vi "move-and-measure_v1.vi"(0 "meter-visa":refnum<visa-resource-name>, 1 "XY-in":dbl[](array[numeric]), 2 "bar-note":u8, 5 "PD Values":cluster{"PD1":dbl, "PD2":dbl, "PD3":dbl}, 7 "stage-refs":T1, 9 "meter-error-in":errorcluster, 11 "stage-error-in":errorcluster, 12 "counter-in":dbl format="%#_13g", 13 "meas#":dbl) -> (3 "measured-point out":dbl[](array[numeric]), 4 "logfile-line-out":string, 6 "iCorr-out":dbl, 10 "meter-error-out":errorcluster, 14 "counter-out":dbl, 15 "stage-error-out":errorcluster)   [LabVIEW 2024]
uses:
  C:/Users/hpDIRC/Desktop/eic_dirc_daq-LabVIEW_new/Thorlabs.MotionControl.IntegratedStepperMotorsCLI.dll
  Thorlabs.MotionControl.IntegratedStepperMotorsCLI.dll
  C:/Users/hpDIRC/Desktop/eic_dirc_daq-LabVIEW_new/Thorlabs.MotionControl.Benchtop.StepperMotorCLI.dll
  Thorlabs.MotionControl.Benchtop.StepperMotorCLI.dll
panel:
  in  "nSamples":dbl=10.0 caption="# Samples"
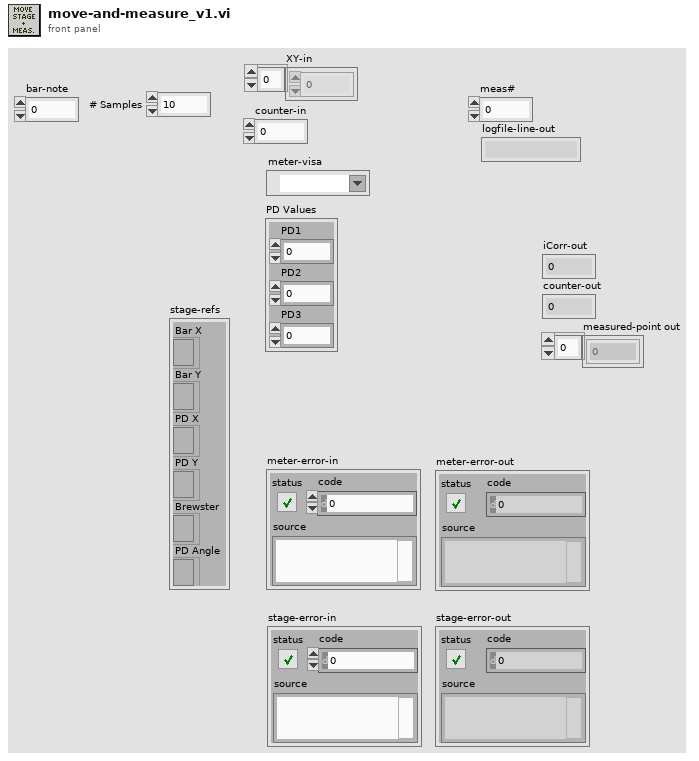
[diagram p1: front panel]
types:
  T1 = cluster{"Bar X":refnum<k24>, "Bar Y":refnum<k24>, "PD X":refnum<k24>, "PD Y":refnum<k24>, "Brewster":refnum<k24>, "PD Angle":refnum<k24>}
  T2 = cluster{"Bar X":dbl, "Bar Y":dbl, "PD X":dbl, "PD Y":dbl, "BMA":dbl, "PDA":dbl}
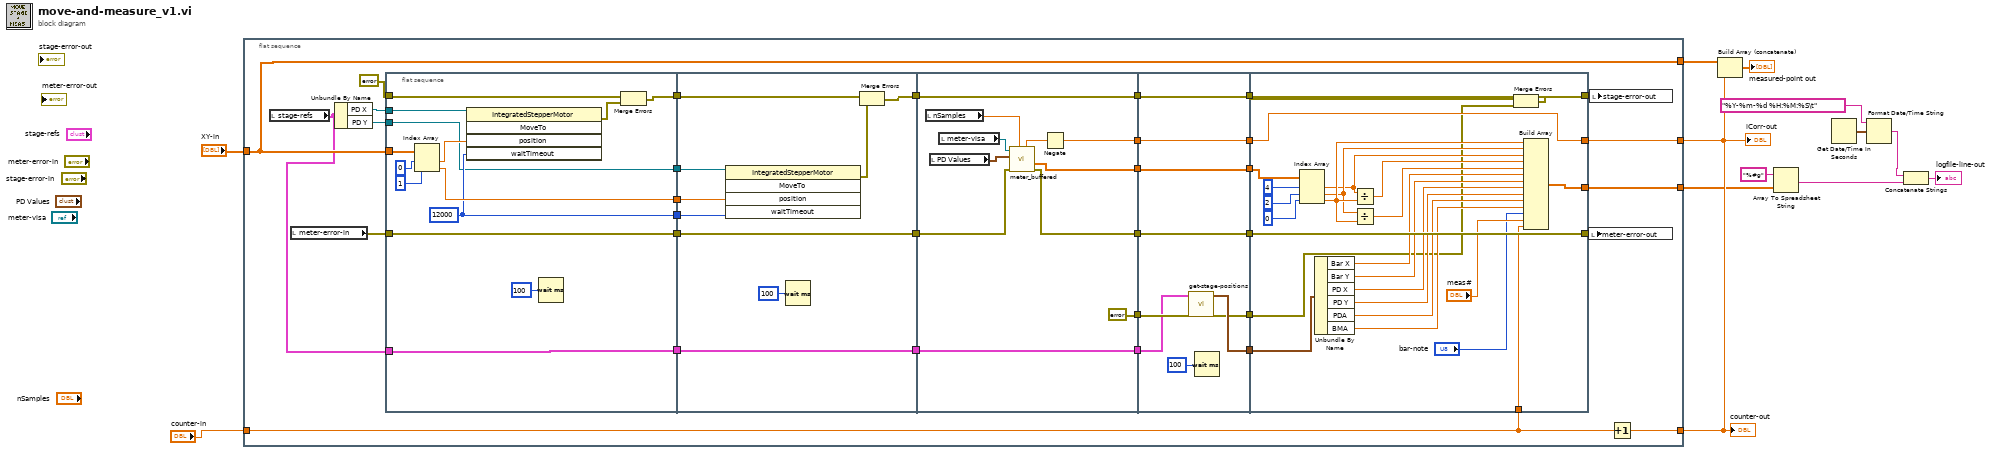
[diagram p0: block diagram]
diagram:
  n1 = flat-sequence {
    tunnel: [w45] -> w9
    tunnel: "XY-in" -> [w41]
    tunnel: "counter-in" -> [w38]
    tunnel: [w39] -> w8
    tunnel: [w41] -> w10
    tunnel: [w37] -> w5
    frame #0 {
      n2 = local read "stage-refs"() -> (w40:T1)
      n3 = local read "meter-error-in"() -> (w42:errorcluster)
      n4 = Unbundle By Name(w40) -> ("PD X"=w46:refnum<k24>, "PD Y"=w16:refnum<k24>)
      n5 = flat-sequence {
        tunnel: w46 -> [w59]
        tunnel: errorcluster {"status"=FALSE, "code"=0, "source"=""} ("stage-error-in") -> [w55]
        tunnel: w41 -> [w53]
        tunnel: w42 -> [w52]
        tunnel: [w54] -> w24
        tunnel: [w52] -> w22
        tunnel: [w51] -> w20
        tunnel: w40 -> [w51]
        tunnel: [w50] -> w18
        tunnel: [w49] -> w17
        tunnel: w16 -> [w48]
        tunnel: [w48] -> w15
        tunnel: w24 -> [w69]
        tunnel: [w63] -> w23
        tunnel: w22 -> [w68]
        tunnel: [w68] -> w21
        tunnel: w20 -> [w67]
        tunnel: [w67] -> w19
        tunnel: w18 -> [w66]
        tunnel: w17 -> [w65]
        tunnel: w15 -> [w64]
        tunnel: w23 -> [w71]
        tunnel: w21 -> [w79]
        tunnel: [w74] -> w36
        tunnel: [w78] -> w34
        tunnel: [w71] -> w32
        tunnel: [w73] -> w30
        tunnel: [w72] -> w28
        tunnel: w19 -> [w72]
        tunnel: [errorcluster {"status"=FALSE, "code"=0, "source"=""} ("error IO")] -> w26
        tunnel: w36 -> [w89]
        tunnel: [w89] -> w35
        tunnel: w34 -> [w88]
        tunnel: [w88] -> w33
        tunnel: w32 -> [w87]
        tunnel: [w87] -> w31
        tunnel: w30 -> [w86]
        tunnel: [w86] -> w29
        tunnel: w28 -> [w81]
        tunnel: [w83] -> w27
        tunnel: w26 -> [w85]
        tunnel: [w82] -> w25
        tunnel: [w91] -> w43
        tunnel: [w114] -> w44
        tunnel: [w96] -> w45
        tunnel: w35 -> [w96]
        tunnel: w33 -> [w114]
        tunnel: w31 -> [w90]
        tunnel: w29 -> [w110]
        tunnel: w27 -> [w93]
        tunnel: w25 -> [w92]
        tunnel: w38 -> [w101]
        tunnel: [w99] -> w37
        frame #0 {
          w49 = 12000 ("waitTimeout")
          n6 = Index Array(array=w53, index #1=0 ("index"), index #2=1 ("index")) -> (element #1=w56:dbl, element #2=w50:dbl)
          n7 = invoke class="IntegratedStepperMotor" method="MoveTo"(reference=w59, "position"=w56, "waitTimeout"=w49) -> (error out=w60:errorcluster)  [unwired: 2 in, 4 out]
          n8 = Wait (ms)(milliseconds to wait=u32 100) -> ()  [unwired: 1 out]
          n9 = Merge Errors(w55, w60) -> (w54:errorcluster)
        }
        frame #1 {
          n10 = invoke class="IntegratedStepperMotor" method="MoveTo"(reference=w64, "position"=w66, "waitTimeout"=w65) -> (error out=w62:errorcluster)  [unwired: 2 in, 4 out]
          n11 = Wait (ms)(milliseconds to wait=u32 100) -> ()  [unwired: 1 out]
          n12 = Merge Errors(w69, w62) -> (w63:errorcluster)
        }
        frame #2 {
          n13 = local read "nSamples"() -> (w77:dbl)
          n14 = local read "PD Values"() -> (w75:cluster{"PD1":dbl, "PD2":dbl, "PD3":dbl})
          n15 = local read "meter-visa"() -> (w76:refnum<visa-resource-name>)
          n16 = call "meter_buffered.vi"("Samples"=w77, "error in"=w79, "PD ranges"=w75, "meter-VISA"=w76) -> ("error out"=w78:errorcluster, "stats-out"=w73:dbl[], "iCorr"=w80:dbl)  [unwired: 3 in, 2 out]
          n17 = Negate(x=w80) -> (-x=w74:dbl)
        }
        frame #3 {
          n18 = call "get-stage-positions.vi"("error in (no error)"=w85, "Cluster"=w81) -> ("error out"=w82:errorcluster, "stage positions"=w83:T2)  [unwired: 8 in]
          n19 = Wait (ms)(milliseconds to wait=u32 100) -> ()  [unwired: 1 out]
        }
        frame #4 {
          n20 = Index Array(array=w110, index #1=4 ("index"), index #2=2 ("index"), index #3=0 ("index")) -> (element #1=w95:dbl, element #2=w97:dbl, element #3=w98:dbl)
          n21 = Unbundle By Name(w93) -> ("Bar X"=w107:dbl, "Bar Y"=w106:dbl, "PD X"=w105:dbl, "PD Y"=w104:dbl, "PDA"=w103:dbl, "BMA"=w102:dbl)
          n22 = Divide(x=w95, y=w98) -> (x/y=w109:dbl)
          n23 = Divide(x=w97, y=w98) -> (x/y=w108:dbl)
          n24 = Merge Errors(w90, w92) -> (w91:errorcluster)
          n25 = Build Array(w98, w97, w95, w109, w108, w107, w106, w105, w104, w103, w102, "bar-note", "meas#", w101) -> (w99:dbl[])
        }
      }
      n26 = local write "meter-error-out"(w44) -> ()
      n27 = local write "stage-error-out"(w43) -> ()
      n28 = Increment(x=w38) -> (x+1=w39:dbl)
    }
  }
  n29 = Build Array (concatenate)(w10, w9, w8) -> (→"measured-point out":dbl[])
  n30 = Array To Spreadsheet String(array=w5, 3:"%#g" ("format string")) -> (spreadsheet string=w3:string)  [unwired: 1 in]
  n31 = Get Date/Time In Seconds() -> (seconds since 1Jan1904=w7:timestamp)
  n32 = Format Date/Time String(time format string (%c)="%Y-%m-%d %H:%M:%S\t", seconds (now)=w7) -> (date/time string=w2:string)  [unwired: 1 in]
  n33 = Concatenate Strings(w2, w3) -> (→"logfile-line-out":string)
  "iCorr-out" <- w9
  "counter-out" <- w8
